vi "SP Calculate TXX.vi"(10 "SP Array (SXX, SXY, SYX, SYY)":cdb[](array[numeric])) -> (2 "TXX":cdb)   [LabVIEW 2011]
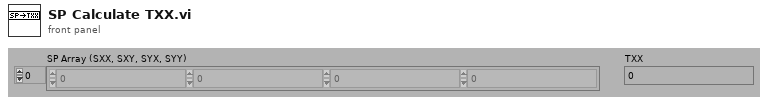
[diagram p1: front panel]
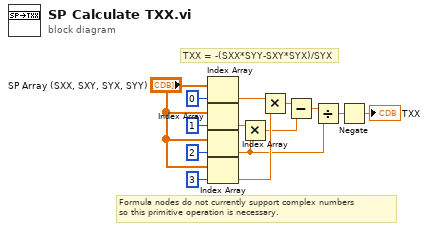
[diagram p0: block diagram]
diagram:
  # "TXX = -(SXX*SYY-SXY*SYX)/SYX"
  # "Formula nodes do not currently support complex numbers\nso this primitive operation is necessary."
  n1 = Index Array(array="SP Array (SXX, SXY, SYX, SYY)", index=0) -> (element=w9:cdb)
  n2 = Index Array(array="SP Array (SXX, SXY, SYX, SYY)", index=1) -> (element=w7:cdb)
  n3 = Index Array(array="SP Array (SXX, SXY, SYX, SYY)", index=2) -> (element=w4:cdb)
  n4 = Index Array(array="SP Array (SXX, SXY, SYX, SYY)", index=3) -> (element=w8:cdb)
  n5 = Multiply(x=w7, y=w4) -> (x*y=w5:cdb)
  n6 = Multiply(x=w9, y=w8) -> (x*y=w6:cdb)
  n7 = Subtract(x=w6, y=w5) -> (x-y=w3:cdb)
  n8 = Divide(x=w3, y=w4) -> (x/y=w2:cdb)
  n9 = Negate(x=w2) -> (-x=→"TXX":cdb)
